vi "InputCalculation.vi"(0 "System no.":i32=1 min=1 max=4 step=1, 5 "error in":errorcluster) -> (14 "Controller error":bool, 19 "error out":errorcluster)   [LabVIEW 2014]
doc: "This VI allows to set the input calculation of the fast alignment input channel.\nFor more information, please refer to the online help of the SIC and SIC? command"
panel:
  in  "Calculation type":i32
  in  "Analog input ID":i32=1 min=1 max=10 step=1
  in  "Set Input Calculation":bool
  in  "Signal input calculation parameters":dbl[](array[numeric])
  in  "stop":bool
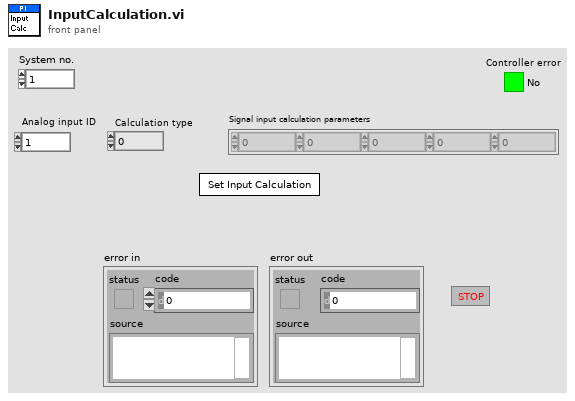
[diagram p1: front panel]
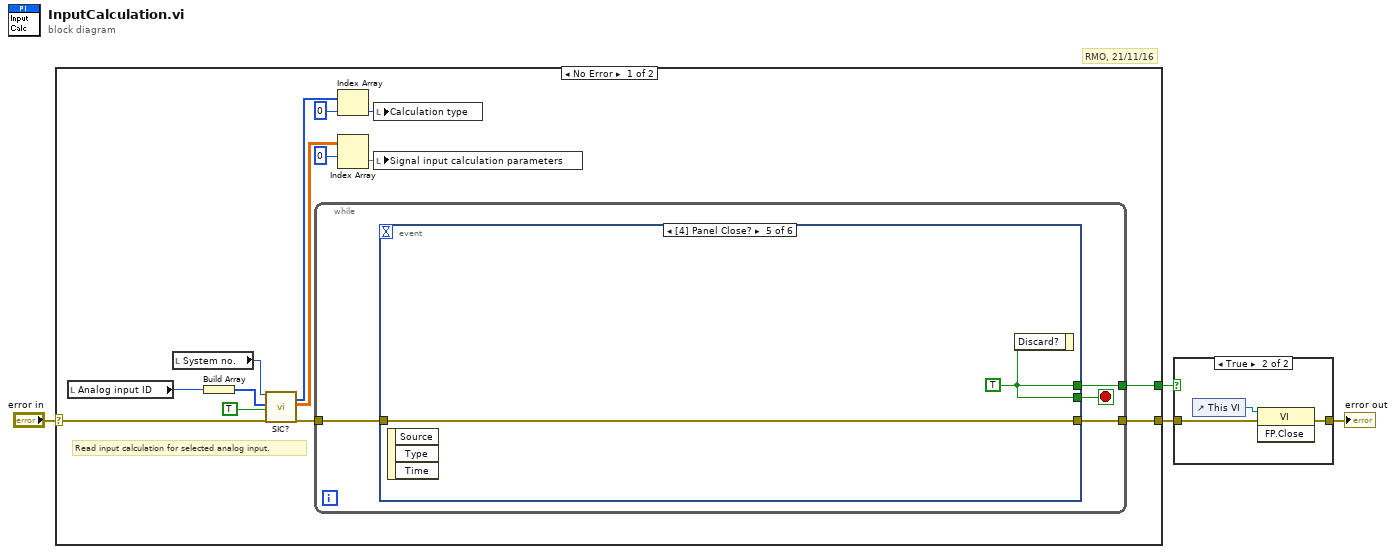
[diagram p0: block diagram]
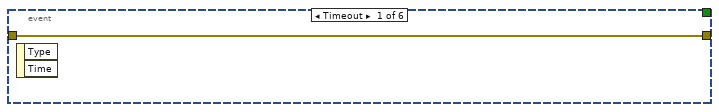
[diagram p3: hidden frame]
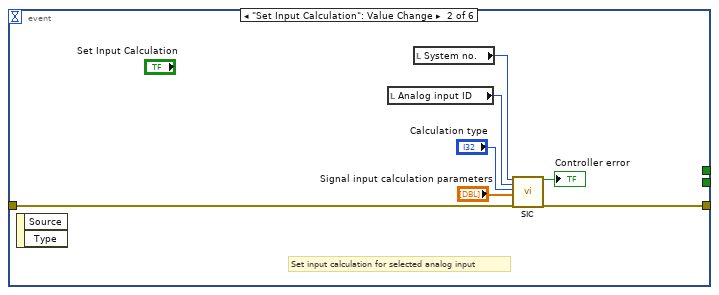
[diagram p4: hidden frame]
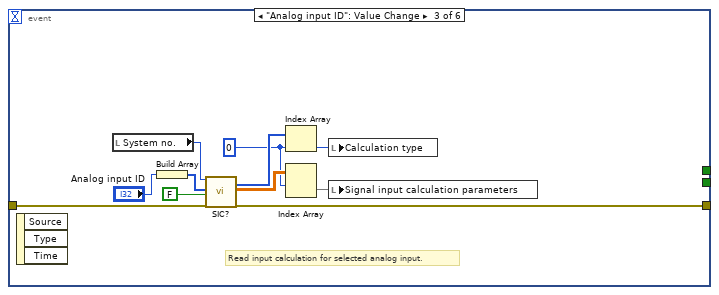
[diagram p5: hidden frame]
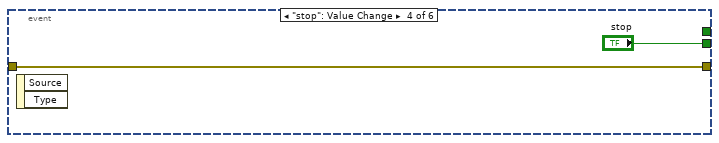
[diagram p6: hidden frame]
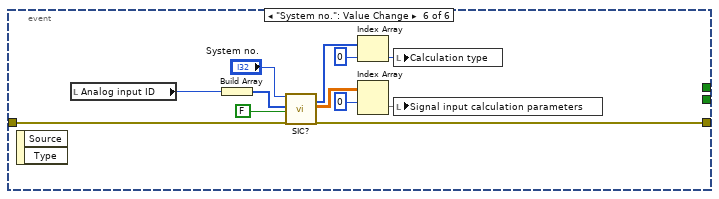
[diagram p7: hidden frame]
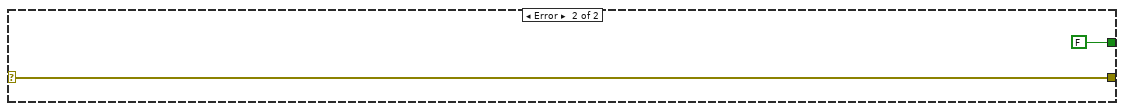
[diagram p8: hidden frame]
diagram:
  # "RMO, 21/11/16"
  n1 = case shown="No Error" "error in" {
    selector: "error in" -> [w17 w59]
    tunnel: [w18 w59] -> w2
    tunnel: [w5 FALSE] -> w3
    frame No Error {
      # "Read input calculation for selected analog input."
      n2 = local read "Analog input ID"() -> (w13:i32)
      n3 = local read "System no."() -> (w15:i32)
      n4 = Build Array(w13) -> (w12:i32[])
      n5 = call "SIC?.vi"("System no."=w15, "Analog input IDs"=w12, "All inputs?"=TRUE, "error in"=w17) -> ("Signal input calculation type"=w11:i32[], "Signal input calculation parameters"=w8:dbl[][], "error out"=w16:errorcluster)  [unwired: 13 out]
      n6 = while {
        tunnel: w16 -> [w21]
        tunnel: [w20] -> w18
        tunnel: [w19] -> w5
        stop <- w22 stop-if-true
        n7 = event shown="[4] Panel Close?" {
          selector: _ -> [_ _ _ _ _ _]
          dyn-events: _ -> [_ _ _ _ _ _]
          timeout: _ -> [_ _ _ _ _ _]
          tunnel: [_ _ _ "stop" w45 _] -> w22
          tunnel: w21 -> [w23 w29 w39 w42 w44 w56]
          tunnel: [w23 w28 w38 w42 w44 w54] -> w20
          tunnel: [_ _ _ _ w45 _] -> w19
          event Timeout {
            n8 = event-data() -> ()  [unwired: 3 out]
          }
          event "Set Input Calculation": Value Change {
            # "Set input calculation for selected analog input"
            n9 = event-data() -> ()  [unwired: 3 out]
            n10 = local read "Analog input ID"() -> (w24:i32)
            n11 = local read "System no."() -> (w30:i32)
            n12 = call "SIC.vi"("System no."=w30, "Analog input ID"=w24, "Calculation type"="Calculation type", "Parameter"="Signal input calculation parameters", "error in"=w29) -> ("Controller error"=→"Controller error":bool, "error out"=w28:errorcluster)  [unwired: 1 in, 12 out]
          }
          event "Analog input ID": Value Change {
            w32 = 0
            # "Read input calculation for selected analog input."
            n13 = event-data() -> ()  [unwired: 4 out]
            n14 = local read "System no."() -> (w40:i32)
            n15 = Build Array("Analog input ID") -> (w36:i32[])
            n16 = call "SIC?.vi"("System no."=w40, "Analog input IDs"=w36, "All inputs?"=FALSE, "error in"=w39) -> ("Signal input calculation type"=w35:i32[], "Signal input calculation parameters"=w33:dbl[][], "error out"=w38:errorcluster)  [unwired: 13 out]
            n17 = Index Array(array=w35, index=w32) -> (element=w34:i32)
            n18 = Index Array(array=w33, index (row)=w32) -> (element=w31:dbl[])  [unwired: 1 in]
            n19 = local write "Calculation type"(w34) -> ()
            n20 = local write "Signal input calculation parameters"(w31) -> ()
          }
          event "stop": Value Change {
            n21 = event-data() -> ()  [unwired: 3 out]
          }
          event Panel Close? {
            w45 = TRUE
            n22 = event-data() -> ()  [unwired: 4 out]
            n23 = event-data("Discard?"=w45) -> ()  [unwired: 1 in, 1 out]
          }
          event "System no.": Value Change {
            n24 = event-data() -> ()  [unwired: 3 out]
            n25 = local read "Analog input ID"() -> (w53:i32)
            n26 = Build Array(w53) -> (w52:i32[])
            n27 = call "SIC?.vi"("System no."="System no.", "Analog input IDs"=w52, "All inputs?"=FALSE, "error in"=w56) -> ("Signal input calculation type"=w47:i32[], "Signal input calculation parameters"=w46:dbl[][], "error out"=w54:errorcluster)  [unwired: 13 out]
            n28 = Index Array(array=w47, index=0) -> (element=w49:i32)
            n29 = Index Array(array=w46, index (row)=0) -> (element=w51:dbl[])  [unwired: 1 in]
            n30 = local write "Calculation type"(w49) -> ()
            n31 = local write "Signal input calculation parameters"(w51) -> ()
          }
        }
      }
      n32 = Index Array(array=w11, index=0) -> (element=w9:i32)
      n33 = Index Array(array=w8, index (row)=0) -> (element=w6:dbl[])  [unwired: 1 in]
      n34 = local write "Calculation type"(w9) -> ()
      n35 = local write "Signal input calculation parameters"(w6) -> ()
    }
    frame Error {
    }
  }
  n36 = case shown="True" w3 {
    tunnel: w2 -> [w60 w62]
    tunnel: [w60 w61] -> w1
    frame False {
    }
    frame True {
      n37 = control-ref of="This VI"() -> (w63:refnum<vi>)
      n38 = invoke class="VI" method="FP.Close"(reference=w63, error in=w62) -> (error out=w61:errorcluster)  [unwired: 1 in, 2 out]
    }
  }
  "error out" <- w1
